vi "Control - Generic - Min Speed Governor Host.vi"() -> ()   [LabVIEW 2015, in "ECS-Host.lvlib"]
uses:
  ECS-Host.lvlib
  <vilib>/addons/Software Calibration Management/XControls/TBL1D.xctl
panel:
  out "PedalOut":sgl caption="[]"
  out "PedalIn":sgl caption="[%]"
  out "PID_DEffort":sgl caption="[]"
  out "PID_IEffort":sgl caption="[]"
  out "PID_PEffort":sgl caption="[]"
  in  "PID_IntMin":sgl caption="[]"
  in  "PID_IntMax":sgl caption="[]"
  in  "PID_DerMin":sgl caption="[]"
  in  "PID_DerMax":sgl caption="[]"
  out "PID_Out":sgl caption="[]"
  in  "PID_Kd":sgl caption="[]"
  in  "PID_Min":sgl caption="[]"
  in  "PID_Max":sgl caption="[]"
  in  "PID_Ki":sgl caption="[%-sec/RPM]"
  in  "PID_Kp":sgl caption="[%/RPM]"
  in  "IdleSpeed_ManE":bool
  in  "IdleSpeed_Man":sgl caption="[RPM]"
  out "IdleSpeed_TblOut":sgl caption="[RPM]"
  in  "PID_E":bool
  in  "IdleSpeed_Tbl":cluster{"X":sgl[], "Y":sgl[]}(xcontrol)
  # "[C]"
  # "[RPM]"
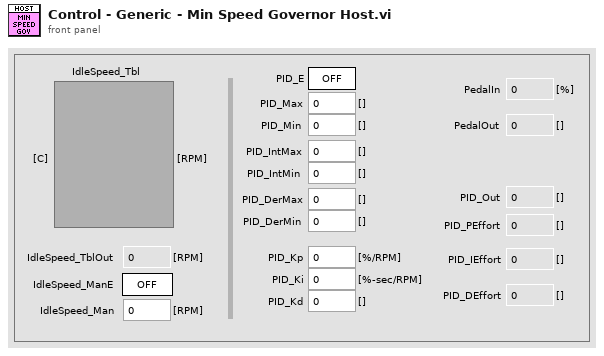
[diagram p1: front panel]
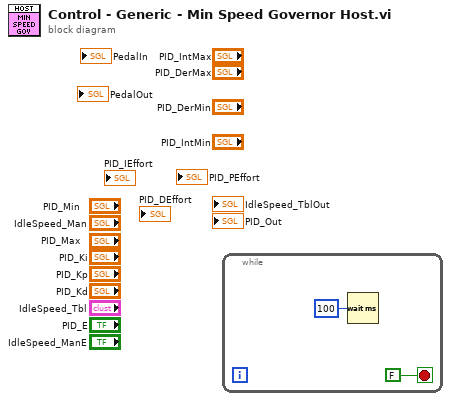
[diagram p0: block diagram]
diagram:
  n1 = while {
    stop <- FALSE stop-if-true
    n2 = Wait (ms)(milliseconds to wait=u32 100) -> ()  [unwired: 1 out]
  }
